vi "GT Get Clock High Precision.vi"(8 "error in (no error)":errorcluster caption="错误输入（无错误）", 10 "pClock":u32, 11 "cardNum":i16) -> (0 "error out":errorcluster caption="错误输出", 2 "pClock out":u32, 3 "function return":i16)   [LabVIEW 2014, in "gts.lvlib"]
doc: "GT_API GT_GetClockHighPrecision(short cardNum,unsigned long *pClock);"
uses:
  gts.lvlib
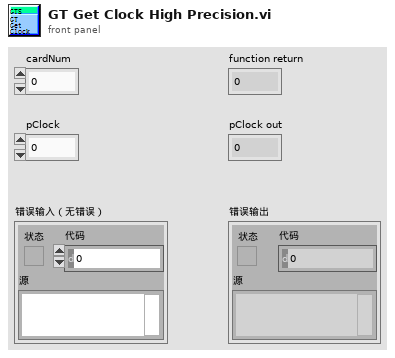
[diagram p1: front panel]
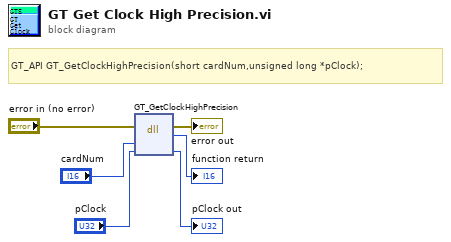
[diagram p0: block diagram]
diagram:
  # "GT_API GT_GetClockHighPrecision(short cardNum,unsigned long *pClock);"
  n1 = dll-call lib="PTH2habs D固高科技资料GTS控制卡GTS卡18年上半年资料dllVC32bit\nmulti_cardgts.*" fn="GT_GetClockHighPrecision"(error in="error in (no error)", "cardNum"="cardNum", "pClock"="pClock") -> (error out=→"error out":errorcluster, →"function return":i16, "pClock"=→"pClock out":u32)  [unwired: 3 in, 1 out]
